vi "Write CellData.vi"(8 "error in":errorcluster, 10 "CellData":refnum<class "PAS Cell Data.lvclass">[](array[class]), 11 "PAS Data in":refnum<class "PAS Data.lvclass">) -> (0 "error out":errorcluster, 3 "PAS Data out":refnum<class "PAS Data.lvclass">)   [LabVIEW 2015, in "PAS Data.lvclass"]
uses:
  PAS Data.lvclass
  Cell/PAS Cell Data.lvclass
  PAS Data.lvclass/PAS Data.ctl
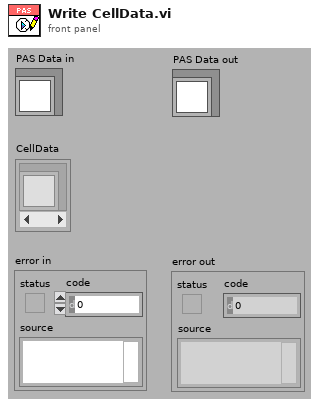
[diagram p1: front panel]
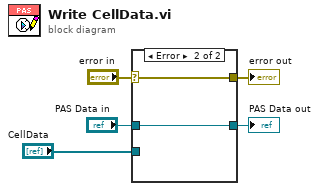
[diagram p0: block diagram]
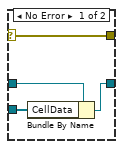
[diagram p2: hidden frame]
diagram:
  n1 = case shown="Error" "error in" {
    selector: "error in" -> [w6 w11]
    tunnel: "PAS Data in" -> [w9 w10]
    tunnel: [w8 w10] -> w4
    tunnel: "CellData" -> [w7 _]
    tunnel: [w6 w11] -> w1
    frame No Error {
      n2 = Bundle By Name(cluster=w9, "CellData"=w7) -> (w8:refnum<class "PAS Data.lvclass">)
    }
    frame Error {
    }
  }
  "error out" <- w1
  "PAS Data out" <- w4
